vi "Scale Corrections.vi"(4 "Compteur":u32, 8 "Bal_in":dbl=0.085 format="%.4f", 9 "Period":u32, 10 "Buoyancy Correction":T1={"Restriction"="3.75", "Bone Dry"=7.001999855041504, "Energie"=7, "Volume"=7.0, "IMC"=70.16566993034309, "Tamb"=70.16566993034309} {"Bone Dry" format="%.2f"}, 11 "Data In":dbl[](array[numeric]) format="%.2f") -> (0 "Bal_out":dbl=0.085 format="%.4f", 1 "ColorW":bool, 3 "Corrected Weight":dbl format="%.2f", 5 "Raw Weight":dbl format="%.2f", 6 "Data Out":dbl[](array[numeric]) format="%.2f", 7 "RMC":dbl format="%.2f")   [LabVIEW 2009]
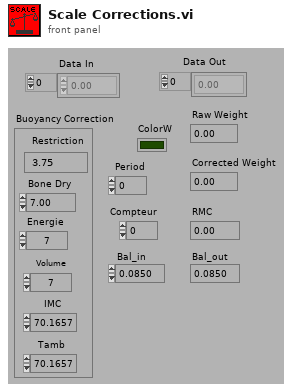
[diagram p1: front panel]
types:
  T1 = cluster{"Restriction":string, "Bone Dry":dbl, "Energie":u8, "Volume":dbl, "IMC":dbl, "Tamb":dbl}
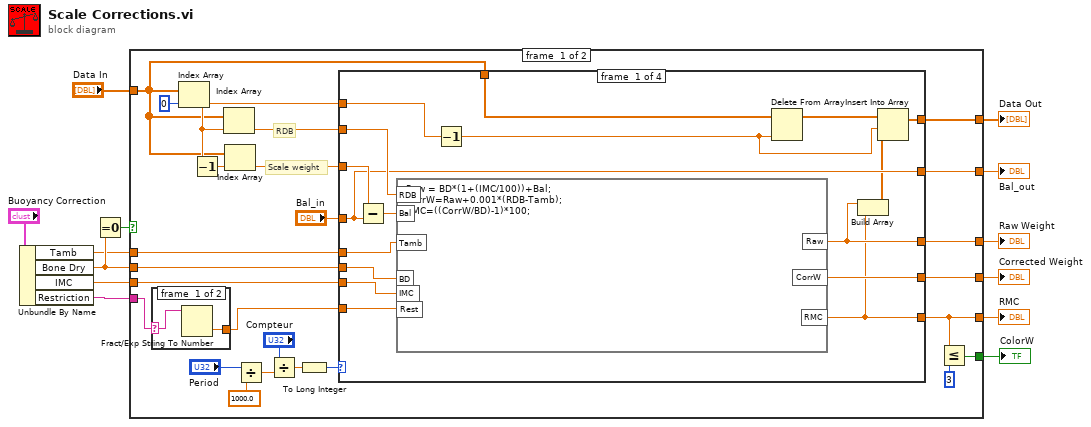
[diagram p0: block diagram]
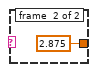
[diagram p2: hidden frame]
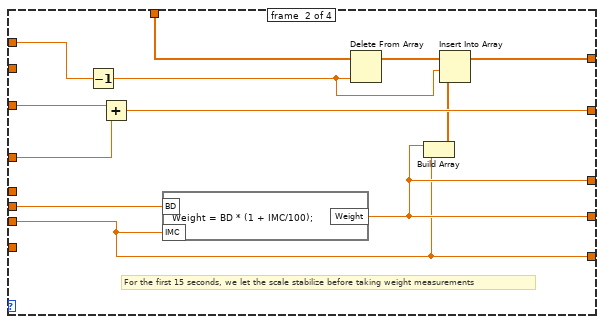
[diagram p3: hidden frame]
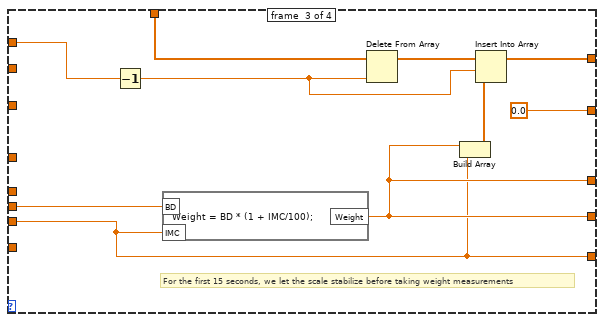
[diagram p4: hidden frame]
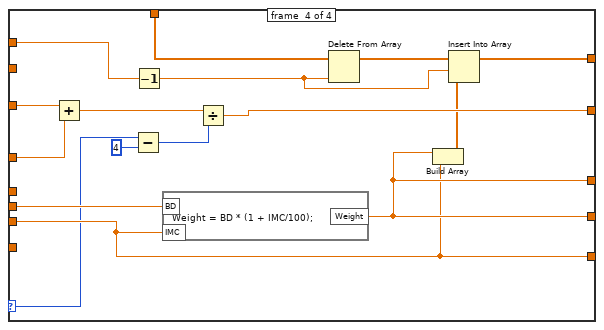
[diagram p5: hidden frame]
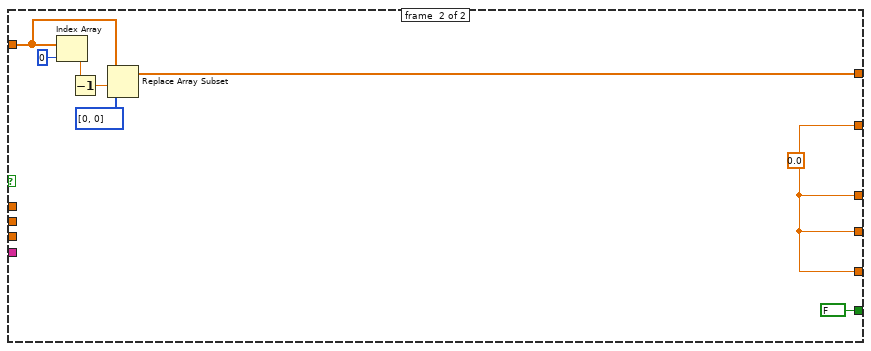
[diagram p6: hidden frame]
diagram:
  n1 = Unbundle By Name("Buoyancy Correction") -> ("Tamb"=w1:dbl, "Bone Dry"=w6:dbl, "IMC"=w5:dbl, "Restriction"=w4:string)
  n2 = Equal To 0?(x=w6) -> (x = 0?=w12:bool)
  n3 = case shown="False" w12 {
    tunnel: [w25 w98] -> w10
    tunnel: [w24 w98] -> w9
    tunnel: [w19 w98] -> w13
    tunnel: "Data In" -> [w23 w102]
    tunnel: [w22 w99] -> w11
    tunnel: [w26 w98] -> w8
    tunnel: w6 -> [w21 _]
    tunnel: w5 -> [w20 _]
    tunnel: w4 -> [w16 _]
    tunnel: [w18 FALSE] -> w3
    tunnel: w1 -> [w14 _]
    frame #0 {
      # "RDB"
      # "Scale weight"
      n4 = case shown="Default" w16 {
        selector: w16 -> [w40 _]
        tunnel: [w39 2.875] -> w15
        frame #0 {
          n5 = Fract/Exp String To Number(string=w40) -> (number=w39:dbl)  [unwired: 3 in, 1 out]
        }
        frame #1 {
        }
      }
      n6 = Index Array(array=w23, index=0 ("Index")) -> (element=w36:dbl)
      n7 = Decrement(x=w36) -> (x-1=w37:dbl)
      n8 = Index Array(array=w23, index=w36) -> (element=w28:dbl)
      n9 = Index Array(array=w23, index=w37) -> (element=w29:dbl)
      n10 = Divide(x="Period", y=1000.0) -> (x/y=w33:dbl)
      n11 = Divide(x="Compteur", y=w33) -> (x/y=w31:dbl)
      n12 = To Long Integer(number=w31) -> (32bit integer=w32:i32)
      n13 = case shown="16, Default" w32 {
        selector: w32 -> [_ _ _ w84]
        tunnel: w29 -> [w53 w70 _ w96]
        tunnel: w28 -> [w55 _ _ _]
        tunnel: "Bal_in" -> [w52 w69 _ w95]
        tunnel: [w52 w68 0.0 ("Bal_in") w91] -> w26
        tunnel: w20 -> [w57 w61 w74 w86]
        tunnel: [w49 w61 w74 w86] -> w19
        tunnel: w21 -> [w58 w67 w80 w94]
        tunnel: w15 -> [w56 _ _ _]
        tunnel: [w50 w62 w75 w87] -> w25
        tunnel: [w51 w62 w75 w87] -> w24
        tunnel: w36 -> [w48 w64 w77 w90]
        tunnel: w23 -> [w47 w65 w78 w89]
        tunnel: [w45 w66 w79 w88] -> w22
        tunnel: w14 -> [w42 _ _ _]
        frame #0 {
          n14 = Subtract(x=w53, y=w52) -> (x-y=w54:dbl)
          n15 = formula code="Raw = BD*(1+(IMC/100))+Bal;\nCorrW=Raw+0.001*(RDB-Tamb);\nRMC=((CorrW/BD)-1)*100;"("Bal"=w54, "BD"=w58, "IMC"=w57, "Rest"=w56, "RDB"=w55, "Tamb"=w42) -> ("Raw"=w50:dbl, "CorrW"=w51:dbl, "RMC"=w49:dbl)
          n16 = Decrement(x=w48) -> (x-1=w43:dbl)
          n17 = Delete From Array(array=w47, index=w43) -> (array with subset deleted=w44:dbl[])  [unwired: 1 in, 1 out]
          n18 = Build Array(w50, w49) -> (w46:dbl[])
          n19 = Insert Into Array(array=w44, index=w43, new element=w46) -> (w45:dbl[])
        }
        frame #1 {
          # "For the first 15 seconds, we let the scale stabilize before taking weight measurements"
          n20 = Decrement(x=w64) -> (x-1=w59:dbl)
          n21 = Add(x=w70, y=w69) -> (x+y=w68:dbl)
          n22 = formula code="Weight = BD * (1 + IMC/100);"("BD"=w67, "IMC"=w61) -> ("Weight"=w62:dbl)
          n23 = Delete From Array(array=w65, index=w59) -> (array with subset deleted=w60:dbl[])  [unwired: 1 in, 1 out]
          n24 = Build Array(w62, w61) -> (w63:dbl[])
          n25 = Insert Into Array(array=w60, index=w59, new element=w63) -> (w66:dbl[])
        }
        frame #2 {
          # "For the first 15 seconds, we let the scale stabilize before taking weight measurements"
          n26 = Decrement(x=w77) -> (x-1=w71:dbl)
          n27 = formula code="Weight = BD * (1 + IMC/100);"("BD"=w80, "IMC"=w74) -> ("Weight"=w75:dbl)
          n28 = Delete From Array(array=w78, index=w71) -> (array with subset deleted=w72:dbl[])  [unwired: 1 in, 1 out]
          n29 = Build Array(w75, w74) -> (w76:dbl[])
          n30 = Insert Into Array(array=w72, index=w71, new element=w76) -> (w79:dbl[])
        }
        frame #3 {
          n31 = Add(x=w96, y=w95) -> (x+y=w93:dbl)
          n32 = Subtract(x=w84, y=4) -> (x-y=w92:i32)
          n33 = Decrement(x=w90) -> (x-1=w81:dbl)
          n34 = formula code="Weight = BD * (1 + IMC/100);"("BD"=w94, "IMC"=w86) -> ("Weight"=w87:dbl)
          n35 = Divide(x=w93, y=w92) -> (x/y=w91:dbl)
          n36 = Delete From Array(array=w89, index=w81) -> (array with subset deleted=w82:dbl[])  [unwired: 1 in, 1 out]
          n37 = Build Array(w87, w86) -> (w85:dbl[])
          n38 = Insert Into Array(array=w82, index=w81, new element=w85) -> (w88:dbl[])
        }
      }
      n39 = Less Or Equal?(x=w19, y=i8 3) -> (x <= y?=w18:bool)
    }
    frame #1 {
      w98 = 0.0
      n40 = Index Array(array=w102, index=0 ("Index")) -> (element=w103:dbl)
      n41 = Decrement(x=w103) -> (x-1=w101:dbl)
      n42 = Replace Array Subset(array=w102, new element=i32[] [0, 0] ("Array Constant"), index=w101) -> (w99:dbl[])
    }
  }
  "RMC" <- w13
  "Corrected Weight" <- w9
  "Raw Weight" <- w10
  "Data Out" <- w11
  "Bal_out" <- w8
  "ColorW" <- w3
